vi "Prepare Config Reload.vi"(8 "error in (no error)":errorcluster, 9 "Reload Options":T1, 11 "Volatus Core in":refnum<class "Volatus Core.lvclass">) -> (0 "error out":errorcluster, 3 "Volatus Core out":refnum<class "Volatus Core.lvclass">)   [LabVIEW 2020, in "Volatus.lvlib" / "Volatus Core.lvclass"]
uses:
  Volatus Core.lvclass
  Reload State.ctl
  Volatus Core.lvclass/Volatus Core.ctl
  Volatus.lvlib
  Config Updater/Config Updater.lvclass
  Reload Options.ctl
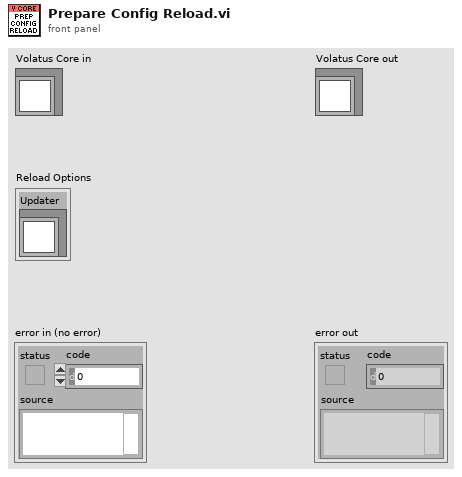
[diagram p1: front panel]
types:
  T1 = typedef "Volatus.lvlib/Reload Options.ctl" = cluster{"Updater":refnum<class "Config Updater.lvclass">}
  T2 = typedef "Volatus.lvlib/Volatus Core.lvclass/Reload State.ctl" = enum16{"None", "Stop Modules", "Close Vecto", "Reload", "Restart"}
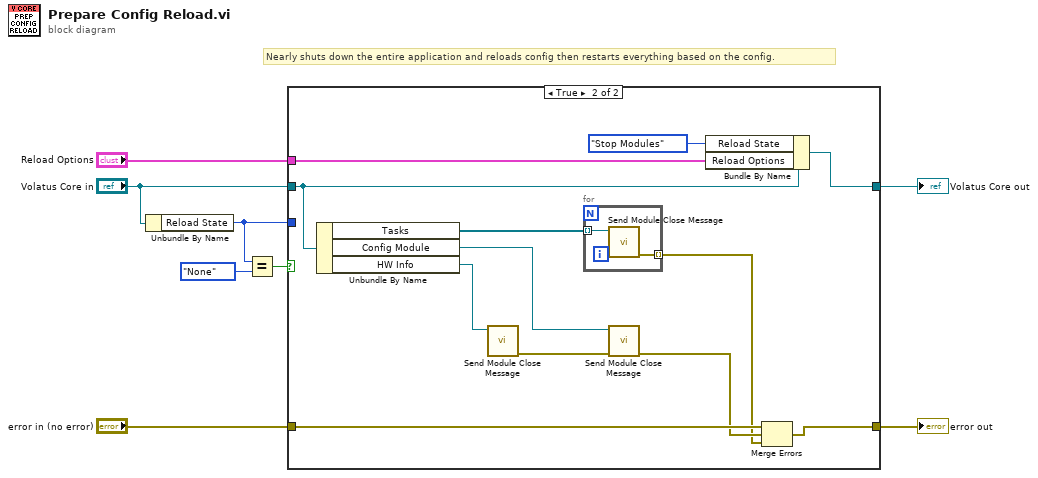
[diagram p0: block diagram]
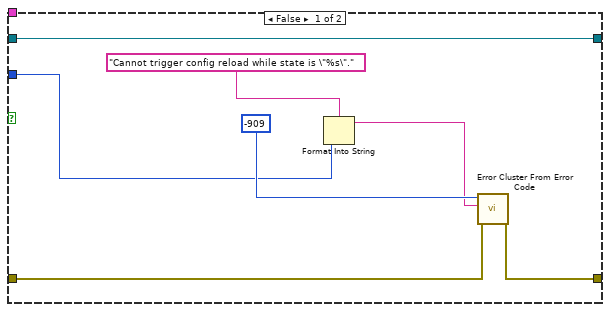
[diagram p2: hidden frame]
diagram:
  # "Nearly shuts down the entire application and reloads config then restarts everything based on the config."
  n1 = Unbundle By Name("Volatus Core in") -> ("Reload State"=w2:T2)
  n2 = Equal?(x=w2, y=Reload_State."None") -> (x = y?=w6:bool)
  n3 = case shown="True" w6 {
    tunnel: "Volatus Core in" -> [w9 w25]
    tunnel: [w9 w20] -> w5
    tunnel: "error in (no error)" -> [w15 w24]
    tunnel: [w14 w21] -> w3
    tunnel: w2 -> [w11 _]
    tunnel: "Reload Options" -> [_ w16]
    frame False {
      n4 = Format Into String(format string="Cannot trigger config reload while state is \"%s\".", w11) -> (resulting string=w10:string)  [unwired: 2 in, 1 out]
      n5 = call <vilib>:"Error Cluster From Error Code.vi"("error in (no error)"=w15, "error message (\"\")"=w10, "error code (0)"=-909) -> ("error out"=w14:errorcluster)  [unwired: 6 in]
    }
    frame True {
      n6 = Unbundle By Name(w25) -> ("Tasks"=w27:refnum<class "MessageQ.lvclass">[], "Config Module"=w26:refnum<class "MessageQ.lvclass">, "HW Info"=w18:refnum<class "MessageQ.lvclass">)
      n7 = call "Send Module Close Message.vi"("MessageQ"=w18) -> ("error out"=w17:errorcluster)  [unwired: 10 in]
      n8 = for {
        tunnel: w27 -> [w29] mode=indexing
        tunnel: [w28] -> w22 mode=indexing
        n9 = call "Send Module Close Message.vi"("MessageQ"=w29) -> ("error out"=w28:errorcluster)  [unwired: 10 in]
      }
      n10 = call "Send Module Close Message.vi"("error in (no error)"=w17, "MessageQ"=w26) -> ("error out"=w23:errorcluster)  [unwired: 9 in]
      n11 = Bundle By Name(cluster=w25, "Reload State"=Reload_State."Stop Modules", "Reload Options"=w16) -> (w20:refnum<class "Volatus Core.lvclass">)
      n12 = Merge Errors(w24, w23, w22) -> (w21:errorcluster)
    }
  }
  "error out" <- w3
  "Volatus Core out" <- w5
